vi "Deploy App.vi"(8 "error in (no error)":errorcluster, 9 "App":refnum<class "ViaApp.lvclass">, 10 "Device":refnum<class "Device.lvclass">, 11 "DeviceDetailPanel in":refnum<class "DeviceDetailPanel.lvclass">) -> (0 "error out":errorcluster, 3 "DeviceDetailPanel out":refnum<class "DeviceDetailPanel.lvclass">)   [LabVIEW 2020, in "PicoG-App.lvlib" / "DeviceDetailPanel.lvclass"]
uses:
  DeviceDetailPanel.lvclass
  ViaApp/ViaApp.lvclass
  Device/Device.lvclass
  Deploy Data.ctl
  DeviceDetailPanel.lvclass/DeviceDetailPanel.ctl
  PicoG-App.lvlib
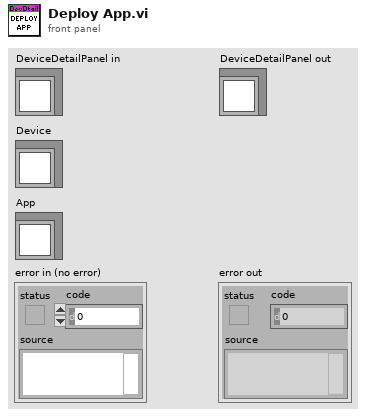
[diagram p1: front panel]
types:
  T1 = typedef "PicoG-App.lvlib/Deploy Data.ctl" = cluster{"App":refnum<class "ViaApp.lvclass">, "Device":refnum<class "Device.lvclass">}
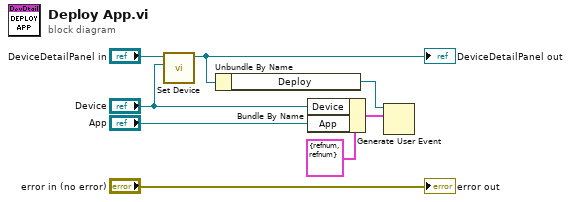
[diagram p0: block diagram]
diagram:
  n1 = call "Set Device.vi"("Device"="Device", "DeviceDetailPanel in"="DeviceDetailPanel in") -> ("DeviceDetailPanel out"=w2:refnum<class "DeviceDetailPanel.lvclass">)  [unwired: 8 in, 1 out]
  "DeviceDetailPanel out" <- w2
  n2 = Unbundle By Name(w2) -> ("Deploy"=w7:refnum<user-event>)
  n3 = Bundle By Name(cluster=T1 {"App"=refnum, "Device"=refnum} ("event data"), "Device"="Device", "App"="App") -> (w5:T1)
  n4 = Generate User Event(user event=w7, event data cluster=w5) -> ()  [unwired: 2 in, 2 out]
  "error out" <- "error in (no error)"
